vi "Sketch.vi"() -> ()   [LabVIEW 2017]
uses:
  <vilib>/myRIO/Instrument Drivers/Onboard IO/DIO/typedefs/DIO Reference.ctl
  <vilib>/myRIO/Common/Instrument Driver Framework/Utilities/typedefs/myRIO Generic Hardware Reference.ctl
  <vilib>/myRIO/Common/Instrument Driver Framework/Utilities/typedefs/Hardware Version Enum.ctl
  <vilib>/myRIO/Common/Instrument Driver Framework/Utilities/typedefs/myRIO v1.0 Reference.ctl
  <vilib>/myRIO/Common/Instrument Driver Framework/Utilities/typedefs/Generic FPGA Reference.ctl
  <vilib>/myRIO/Common/Instrument Driver Framework/myRIO v1.0/DIO/typedefs/DIO Channels List.ctl
  <vilib>/myRIO/Common/Instrument Driver Framework/myRIO v1.0/DIO/typedefs/DIO Channels Enum.ctl
  <vilib>/userdefined/High Color/nirio_resource_hc.ctl
  <vilib>/myRIO/Common/Instrument Driver Framework/myRIO v1.0/DIO/vis/myRIO v1.1 Open DIO.vi
  <vilib>/myRIO/Common/Instrument Driver Framework/Utilities/vis/Validate Channels.vi
  <vilib>/myRIO/Common/Instrument Driver Framework/myRIO v1.0/DIO/vis/myRIO v1.0 Reserve DIO.vi
  <vilib>/myRIO/Common/Instrument Driver Framework/myRIO v1.0/Resource Manager/vis/myRIO v1.0 Reserve Channel List.vi
  <vilib>/myRIO/Common/Instrument Driver Framework/myRIO v1.0/DIO/vis/myRIO v1.0 Build MUX Configuration DIO.vi
  <vilib>/myRIO/Common/Instrument Driver Framework/myRIO v1.0/Resource Manager/vis/myRIO v1.0 Reserve Channel.vi
  <vilib>/myRIO/Common/Instrument Driver Framework/myRIO v1.0/Resource Manager/vis/myRIO v1.0 Unreserve Channel.vi
  <vilib>/myRIO/Common/Instrument Driver Framework/myRIO v1.0/Resource Manager/vis/myRIO v1.0 Create Configuration List.vi
  <vilib>/myRIO/Common/Instrument Driver Framework/myRIO v1.0/Resource Manager/vis/myRIO v1.0 Build Mutex Name.vi
  <vilib>/Utility/VariantDataType/GetNumericInfo.vi
  <vilib>/Utility/error.llb/Error Cluster From Error Code.vi
  <vilib>/myRIO/Common/Instrument Driver Framework/myRIO v1.0/myRIO v1.1 Open.vi
  <vilib>/myRIO/Common/Instrument Driver Framework/Utilities/vis/IO Manager.vi
  <vilib>/myRIO/Common/Instrument Driver Framework/Utilities/vis/Configuration Manager.vi
  <vilib>/myRIO/Common/Instrument Driver Framework/myRIO v1.0/Resource Manager/vis/myRIO v1.0 Configure IO.vi
  <vilib>/myRIO/Common/Instrument Driver Framework/myRIO v1.0/myRIO v1.0 Close.vi
  <vilib>/myRIO/Common/Instrument Driver Framework/myRIO v1.0/DIO/vis/myRIO v1.0 Write DIO.vi
  <vilib>/myRIO/Instrument Drivers/Onboard IO/DIO/vis/myRIO DIO Open.xnode
  <vilib>/myRIO/Instrument Drivers/Onboard IO/DIO/DIO.lvlib
panel:
  in  "milliseconds to wait":u32
  out "Total":i32
  in  "Frequency [Hz]":dbl=50.0
  in  "Duty Cycle":dbl(knob)=0.025 scale=0.025..0.12
  in  "Servo":tag="A/PWM0"
  out "error out":errorcluster
  in  "Step size":T1(ring)
  in  "Microstep":tag[](array[tag])=["C/DIO5", "C/DIO6", "C/DIO7"]
  out "floor(x/y) 2":i32
  in  "stop":bool
  in  "DIO3":tag[](array[tag])=["C/DIO3"]
  in  "Rotation":u16(ring) items=["Half", "Full"]
  in  "Speed":u32=20
  in  "Enable":bool
  in  "DIO2":tag[](array[tag])=["C/DIO2"]
  in  "Step":bool
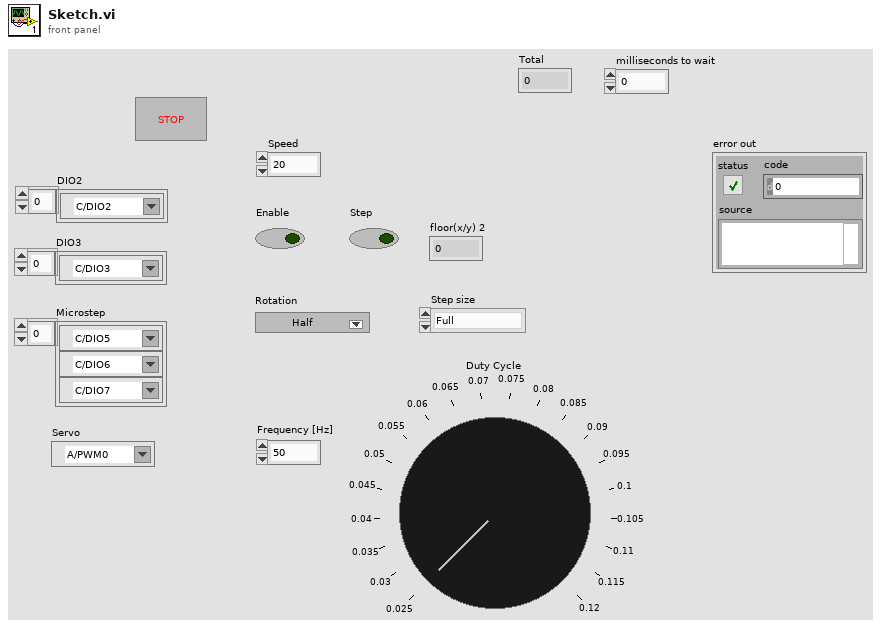
[diagram p1: front panel]
types:
  T1 = enum16{"Full", "Half", "Quarter", "Eighth", "Sixteenth"}
  T2 = typedef "nirio_resource_hc.ctl" = tag
  T3 = typedef "Hardware Version Enum.ctl" = enum16{"Unknown", "myRIO-1900", "myRIO-1950", "roboRIO", "NI ELVIS RIO CM"}
  T4 = typedef "DIO.lvlib/DIO Reference.ctl" = cluster{"myRIO Reference":T5, "DIO Channels List":T8}
  T5 = typedef "myRIO Generic Hardware Reference.ctl" = cluster{"myRIO Model":T3, "myRIO Hardware Reference":T6}
  T6 = typedef "myRIO v1.0 Reference.ctl" = cluster{"Generic FPGA Reference":T7, "Allow multiple opens":bool}
  T7 = typedef "Generic FPGA Reference.ctl" = refnum<k20>
  T8 = typedef "DIO Channels List.ctl" = T9[]
  T9 = typedef "DIO Channels Enum.ctl" = enum16{"Not Connected", "C/DIO0", "C/DIO1", "C/DIO2", "C/DIO3", "C/DIO4", "C/DIO5", "C/DIO6", "C/DIO7", "A/DIO0", "A/DIO1", "A/DIO2", "A/DIO3", "A/DIO4", "A/DIO5", "A/DIO6", "A/DIO7", "A/DIO8", "A/DIO9", "A/DIO10", "A/DIO11", "A/DIO12", "A/DIO13", "A/DIO14", "A/DIO15", "B/DIO0", "B/DIO1", "B/DIO2", "B/DIO3", "B/DIO4", "B/DIO5", "B/DIO6", "B/DIO7", "B/DIO8", "B/DIO9", "B/DIO10", "B/DIO11", "B/DIO12", "B/DIO13", "B/DIO14", "B/DIO15", "LED0", "LED1", "LED2", "LED3", "Button0", "DIO/DIO0", "DIO/DIO1", "DIO/DIO2", "DIO/DIO3", "DIO/DIO4", "DIO/DIO5", "DIO/DIO6", "DIO/DIO7", "DIO/DIO8", "DIO/DIO9", "SPI/CS0", "SPI/CS1", "SPI/CS2", "SPI/CS3", "LED RADIO (Green)", "LED RADIO (Red)", "LED COMM (Green)", "LED COMM (Red)", "LED MODE (Green)", "LED MODE (Red)"}
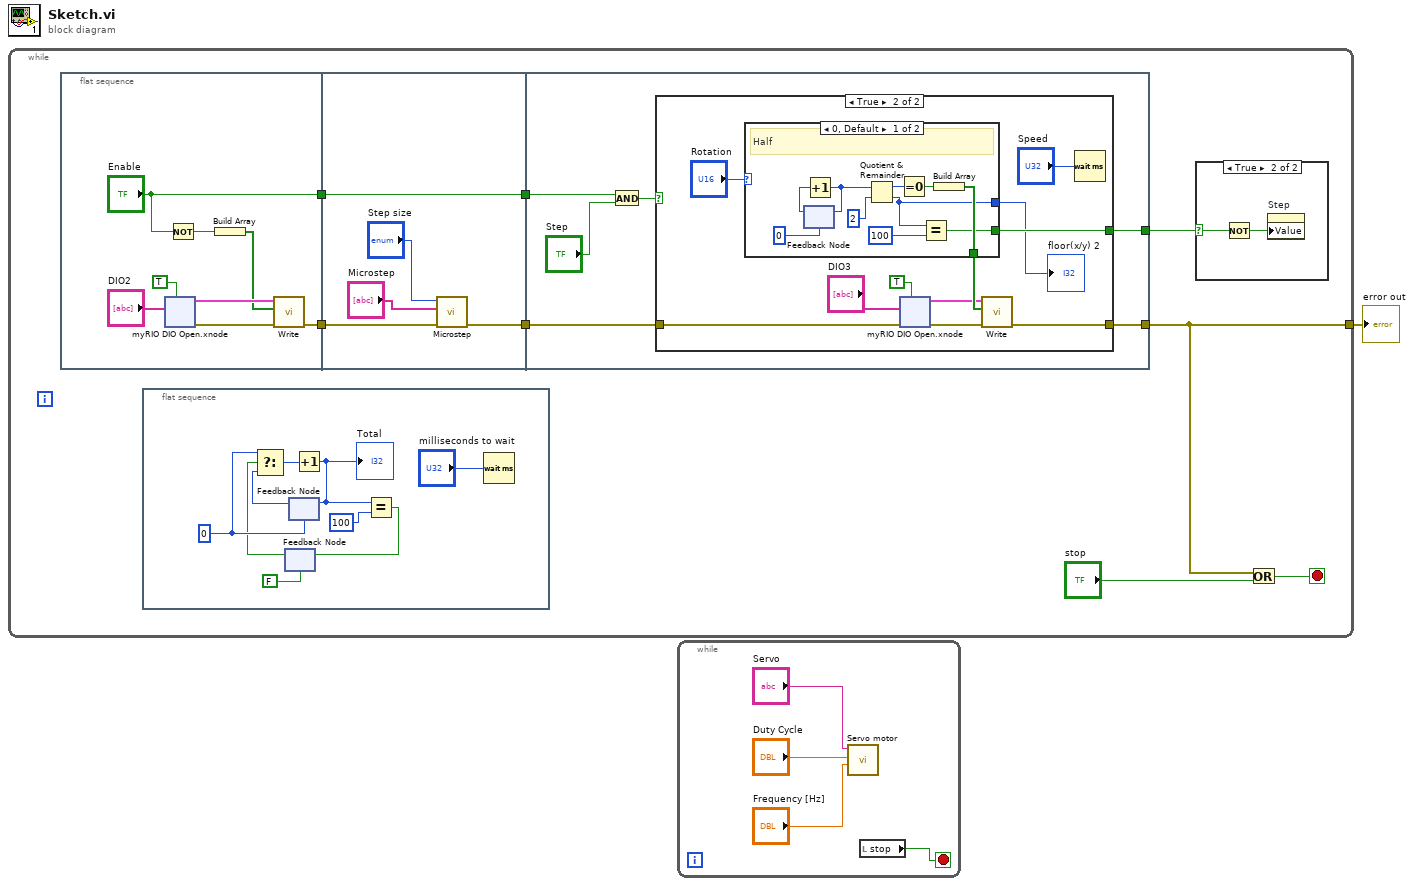
[diagram p0: block diagram]
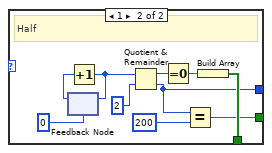
[diagram p4: hidden frame]
diagram:
  n1 = while {
    tunnel: [w3] -> w1
    stop <- w8 stop-if-true
    n2 = flat-sequence {
      tunnel: ["Enable"] -> w7
      tunnel: [w21] -> w5
      tunnel: w7 -> [w49]
      tunnel: [w49] -> w6
      tunnel: w5 -> [w46]
      tunnel: [w45] -> w4
      tunnel: [w55] -> w2
      tunnel: w6 -> [w54]
      tunnel: w4 -> [w51]
      tunnel: [w50] -> w3
      frame #0 {
        n3 = xnode "myRIO DIO Open.xnode"("Allow multiple opens?"=TRUE, "Channel Names"="DIO2") -> ("error out"=w28:errorcluster, "DIO Ref Out"=w27:T4)  [unwired: 1 in]
        n4 = Not(x="Enable") -> (.not. x?=w23:bool)
        n5 = Build Array(w23) -> (w24:bool[])
        n6 = call <vilib>:"Write.vi"("error in (no error)"=w28, "Values"=w24, "DIO Ref In"=w27) -> ("error out"=w21:errorcluster)  [unwired: 6 in, 1 out]
      }
      frame #1 {
        n7 = call "Microstep.vi"("error in (no error)"=w46, "Microstep"="Microstep", "Step size"="Step size") -> ("error out"=w45:errorcluster)  [unwired: 7 in, 1 out]
      }
      frame #2 {
        n8 = And(x=w54, y="Step") -> (x .and. y?=w53:bool)
        n9 = case shown="True" w53 {
          selector: w53 -> [w57 _]
          tunnel: [w57 w61] -> w55
          tunnel: w51 -> [w56 w59]
          tunnel: [w56 w58] -> w50
          frame False {
          }
          frame True {
            n10 = case shown="0, Default" "Rotation" {
              tunnel: [w77 w87] -> w68
              tunnel: [w71 w81] -> w61
              tunnel: [w69 w79] -> w60
              frame 0, Default {
                # "Half"
                n11 = feedback #1(0) -> (w75:i32)
                n12 = Increment(x=w75) -> (x+1=w74:i32)
                n13 = feedback-in #1(w74) -> ()
                n14 = Quotient & Remainder(x=w74, y=2) -> (x-y*floor(x/y)=w78:i32, floor(x/y)=w69:i32)
                n15 = Equal To 0?(x=w78) -> (x = 0?=w76:bool)
                n16 = Equal?(x=w69, y=100) -> (x = y?=w71:bool)
                n17 = Build Array(w76) -> (w77:bool[])
              }
              frame 1 {
                # "Half"
                n18 = feedback #2(0) -> (w85:i32)
                n19 = Increment(x=w85) -> (x+1=w84:i32)
                n20 = feedback-in #2(w84) -> ()
                n21 = Quotient & Remainder(x=w84, y=2) -> (x-y*floor(x/y)=w88:i32, floor(x/y)=w79:i32)
                n22 = Equal To 0?(x=w88) -> (x = 0?=w86:bool)
                n23 = Equal?(x=w79, y=200) -> (x = y?=w81:bool)
                n24 = Build Array(w86) -> (w87:bool[])
              }
            }
            "floor(x/y) 2" <- w60
            n25 = xnode "myRIO DIO Open.xnode"("error in (no error)"=w59, "Allow multiple opens?"=TRUE, "Channel Names"="DIO3") -> ("error out"=w65:errorcluster, "DIO Ref Out"=w66:T4)
            n26 = call <vilib>:"Write.vi"("error in (no error)"=w65, "Values"=w68, "DIO Ref In"=w66) -> ("error out"=w58:errorcluster)  [unwired: 6 in, 1 out]
            n27 = Wait (ms)(milliseconds to wait="Speed") -> ()  [unwired: 1 out]
          }
        }
      }
    }
    n28 = flat-sequence {
      frame #0 {
        w14 = 0
        n29 = feedback #3(FALSE) -> (w12:bool)
        n30 = feedback #4(w14) -> (w15:i32)
        n31 = Select(t=w14, s=w12, f=w15) -> (s? t:f=w16:i32)
        n32 = Increment(x=w16) -> (x+1=w18:i32)
        "Total" <- w18
        n33 = feedback-in #4(w18) -> ()
        n34 = Equal?(x=w18, y=100) -> (x = y?=w13:bool)
        n35 = feedback-in #3(w13) -> ()
        n36 = Wait (ms)(milliseconds to wait="milliseconds to wait") -> ()  [unwired: 1 out]
      }
    }
    n37 = case shown="True" w2 {
      selector: w2 -> [_ w20]
      frame False {
      }
      frame True {
        n38 = Not(x=w20) -> (.not. x?=w19:bool)
        n39 = property on="Step" class="Bool (strict)"("Value"=w19) -> ()  [unwired: 2 in, 2 out]
      }
    }
    n40 = Or(x=w3, y="stop") -> (x .or. y?=w8:bool)
  }
  "error out" <- w1
  n41 = while {
    stop <- w105 stop-if-true
    n42 = call "Servo motor.vi"("Frequency [Hz]"="Frequency [Hz]", "Duty Cycle"="Duty Cycle", "Servo"="Servo") -> ()  [unwired: 7 in, 2 out]
    n43 = local read "stop"() -> (w105:bool)
  }
